vi "Is Valid.vi"(8 "error in (no error)":errorcluster, 11 "CFG JSON Base in":refnum<class "CFG JSON Base.lvclass">) -> (0 "error out":errorcluster, 2 "Is Valid?":bool, 3 "CFG JSON Base out":refnum<class "CFG JSON Base.lvclass">)   [LabVIEW 2023, in "HAL GOOP4.lvlib" / "CFG JSON Base.lvclass"]
uses:
  CFG JSON Base.lvclass
  CFG JSON Base.lvclass/CFG JSON Base.ctl
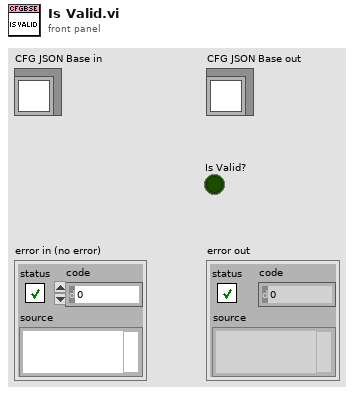
[diagram p1: front panel]
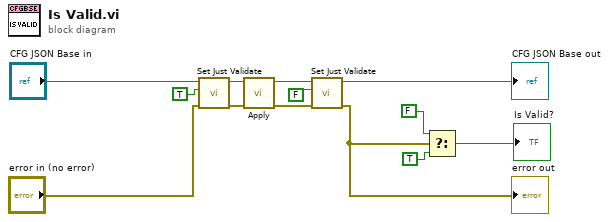
[diagram p0: block diagram]
diagram:
  n1 = call "Set Just Validate.vi"("error in (no error)"="error in (no error)", "Just Validate"=TRUE, "CFG JSON Base in"="CFG JSON Base in") -> ("error out"=w7:errorcluster, "CFG JSON Base out"=w8:refnum<class "CFG JSON Base.lvclass">)  [unwired: 7 in]
  n2 = call-dynamic "Apply.vi"("error in (no error)"=w7, "IConfigure in"=w8) -> ("error out"=w5:errorcluster, "IConfigure out"=w4:refnum<class "CFG JSON Base.lvclass">)  [unwired: 8 in]
  n3 = call "Set Just Validate.vi"("error in (no error)"=w5, "Just Validate"=FALSE, "CFG JSON Base in"=w4) -> ("error out"=w12:errorcluster, "CFG JSON Base out"=→"CFG JSON Base out":refnum<class "CFG JSON Base.lvclass">)  [unwired: 7 in]
  "error out" <- w12
  n4 = Select(t=FALSE, s=w12, f=TRUE) -> (s? t:f=→"Is Valid?":bool)
